vi "未命名 2.vi"() -> ()   [LabVIEW 2018]
panel:
  out "max(x,y)":dbl
  in  "y":dbl
  in  "x":dbl
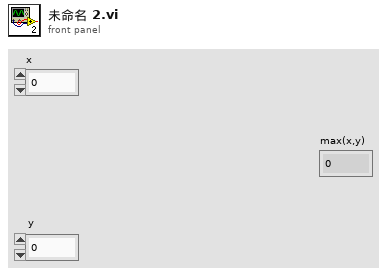
[diagram p1: front panel]
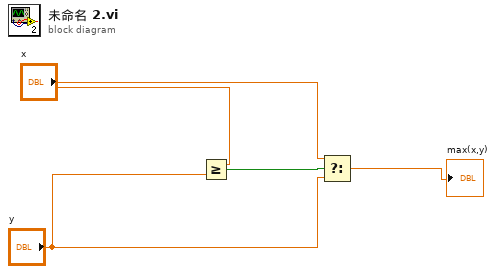
[diagram p0: block diagram]
diagram:
  n1 = Greater Or Equal?(x="x", y="y") -> (x >= y?=w4:bool)
  n2 = Select(t="x", s=w4, f="y") -> (s? t:f=→"max(x,y)":dbl)
